vi "Hadamard.vi"(8 "error in (no error)":errorcluster, 10 "Wire in":T1, 11 "Gate in":refnum<class "G-UE.lvclass">) -> (0 "error out":errorcluster, 3 "Gate out":refnum<class "G-UE.lvclass">)   [LabVIEW 2016, in "G-UE.lvclass"]
uses:
  G-UE.lvclass
  TypeDefs/Circuit Cluster.ctl
  GateAbst/GateAbst.lvclass
  <vilib>/Analysis/Matrix/Datatypes/ComplexMatrix.ctl
  <vilib>/Analysis/Matrix/Numeric/Multiply/Multiply - CM,C.vi
  <vilib>/Analysis/Matrix/NI_Matrix.lvlib
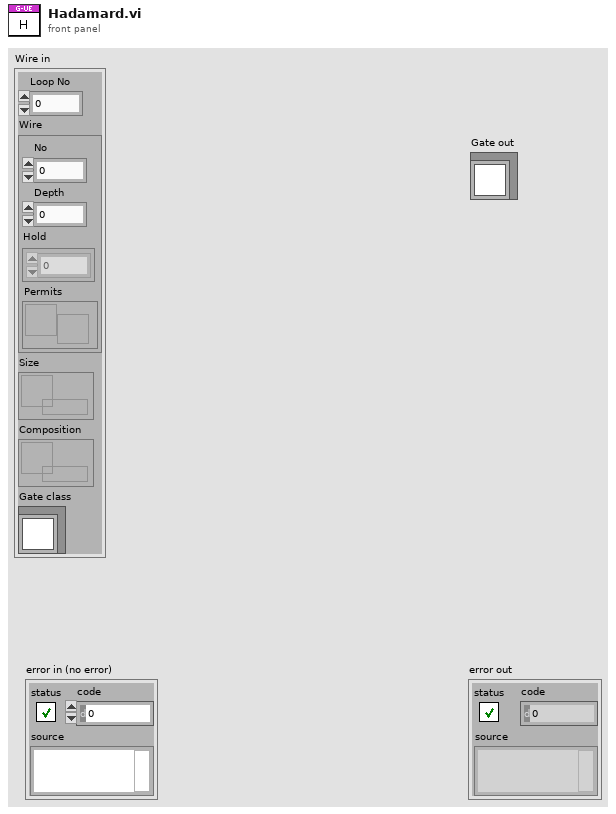
[diagram p1: front panel]
types:
  T1 = typedef "Circuit Cluster.ctl" = cluster{"Loop No":i32, "Wire":cluster{"No":i32, "Depth":i32, "Hold":i32[][], "Permits":refnum<notifier>}, "Size":refnum<queue>, "Composition":refnum<queue>, "Gate class":refnum<class "GateAbst.lvclass">}
  T2 = typedef "NI_Matrix.lvlib/ComplexMatrix.ctl" = cdb[][]
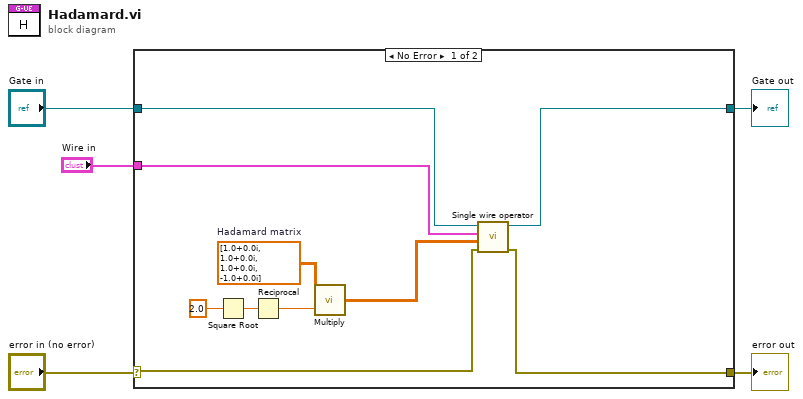
[diagram p0: block diagram]
diagram:
  n1 = case shown="No Error" "error in (no error)" {
    selector: "error in (no error)" -> [w8 w17]
    tunnel: [w7 w17] -> w4
    tunnel: [w9 w16] -> w2
    tunnel: "Gate in" -> [w10 w16]
    tunnel: "Wire in" -> [w6 _]
    frame No Error {
      w15 = T2 [[1.0+0.0i, 1.0+0.0i], [1.0+0.0i, -1.0+0.0i]]  # Hadamard matrix
      n2 = Square Root(x=2.0) -> (sqrt(x)=w12:dbl)
      n3 = Reciprocal(x=w12) -> (1/x=w14:dbl)
      n4 = call-poly <vilib>:"Multiply.vi"("Complex Scalar c"=w14, "Complex Matrix A"=w15) -> ("A * c"=w11:T2)
      n5 = call "Single wire operator.vi"("error in (no error)"=w8, "Operator matrix"=w11, "Wire in"=w6, "G-UE in"=w10) -> ("error out"=w7:errorcluster, "G-UE out"=w9:refnum<class "G-UE.lvclass">)  [unwired: 6 in]
    }
    frame Error {
    }
  }
  "error out" <- w4
  "Gate out" <- w2
